vi "Get Temperature WAV.vi"(8 "error in":errorcluster, 10 "Source":string, 11 "Thermometer Multichannel Worker in":refnum<class "Thermometer Multichannel Worker.lvclass">) -> (0 "error out":errorcluster, 2 "Temperature":waveform(dbl), 3 "Thermometer Multichannel Worker out":refnum<class "Thermometer Multichannel Worker.lvclass">)   [LabVIEW 2024, in "Thermometer Multichannel Worker.lvlib" / "Thermometer Multichannel Worker.lvclass"]
uses:
  Thermometer Multichannel Worker.lvclass
  Thermometer Multichannel Worker.lvclass/Thermometer Multichannel Worker.ctl
  <vilib>/Waveform/WDTOps.llb/WDT Append Waveforms DBL.vi
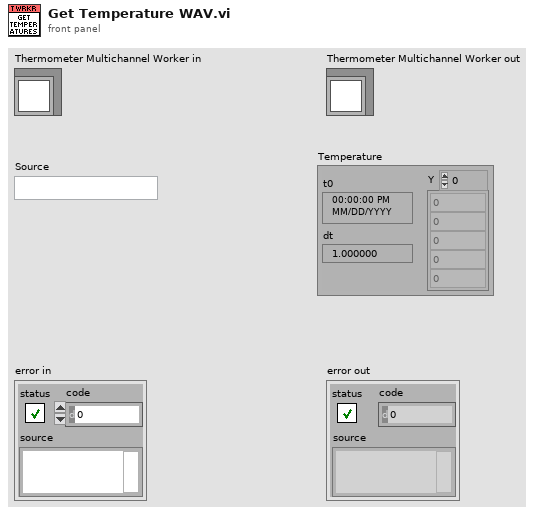
[diagram p1: front panel]
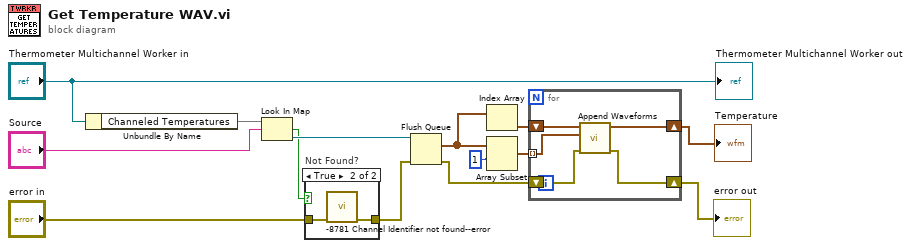
[diagram p0: block diagram]
diagram:
  n1 = Unbundle By Name("Thermometer Multichannel Worker in") -> ("Channeled Temperatures"=w13:map{string, refnum<queue>})
  n2 = Look In Map(map=w13, key="Source") -> (key not found?=w8:bool, value=w11:refnum<queue>)  [unwired: 1 in]
  n3 = case "Not Found?" shown="True" w8 {
    tunnel: [w15 w17] -> w10
    tunnel: "error in" -> [w15 w16]
    frame False {
    }
    frame True {
      n4 = call "-8781 Channel Identifier not found--error.vi"("error in"=w16) -> ("error out"=w17:errorcluster)  [unwired: 10 in]
    }
  }
  n5 = Flush Queue(queue=w11, error in (no error)=w10) -> (remaining elements=w6:waveform(dbl)[], error out=w3:errorcluster)  [unwired: 1 out]
  n6 = Index Array(array=w6) -> (element=w7:waveform(dbl))  [unwired: 1 in]
  n7 = Array Subset(array=w6, index=1) -> (w5:waveform(dbl)[])  [unwired: 1 in]
  n8 = for {
    tunnel: w5 -> [w21] mode=indexing
    shift-right: [w19] -> w2
    shift-left: w3 -> [w20]
    shift-right: [w18] -> w1
    shift-left: w7 -> [w22]
    n9 = call-poly <vilib>:"Append Waveforms.vi"("error in (no error)"=w20, "waveform B"=w21, "waveform A"=w22) -> ("error out"=w19:errorcluster, "waveform out"=w18:waveform(dbl))  [unwired: 7 in]
  }
  "error out" <- w2
  "Temperature" <- w1
  "Thermometer Multichannel Worker out" <- "Thermometer Multichannel Worker in"
